vi "Teleop.vi"(10 "Match Info":T3={"Autonomous Elapsed Seconds"=0.0, "TeleOp Elapsed Seconds"=0.0, "Disabled Elapsed Seconds"=0.0, "Visited Autonomous"=FALSE, "Visited TeleOp"=FALSE, "Visited Disabled"=FALSE, "Autonomous Settings"={"Autonomous Style"=enum."Independent", "VI Refnum"=refnum}}, 11 "Call Context":T4) -> ()   [LabVIEW 2014]
doc: "This VI is called for each TeleOp packet received from the DS where the robot is not disabled. It is often used to read from the joysticks and update I/O or to update setpoints for timed control loops. It should complete and return within 20 milliseconds or it may miss DS packets."
uses:
  <vilib>/Rock Robotics/WPI/DriverStation/WPI_DriverStationDerivedRobotMode.ctl
  <vilib>/Rock Robotics/WPI/DriverStation/WPI_DriverStationMatch Info.ctl
  <vilib>/Rock Robotics/WPI/CAN/TalonSRX/WPI_CANTalonSRX_APIControlMode.ctl
  <vilib>/Rock Robotics/Network Tables/SD Write Boolean.vi
  <vilib>/Rock Robotics/Network Tables/SD Read Boolean.vi
  <vilib>/Rock Robotics/Network Tables/SD Read Number.vi
  <vilib>/Rock Robotics/WPI/Joystick/WPI_JoystickGetSetRefNum.vi
panel:
  out "ej Distance":dbl
  out "ej Rate":dbl
  out "Time elapsed":u64
  in  "Set Timer":bool
  out "cluster":T1
  out "Btm lim val":bool
  out "top lim val":bool
  out "Toggled Boolean":bool
  out "axes":T2
  out "Sample Slider 0":dbl(slide) scale=0.0..5.0
  out "Sample Boolean 1":bool
  out "Sample Boolean 0":bool
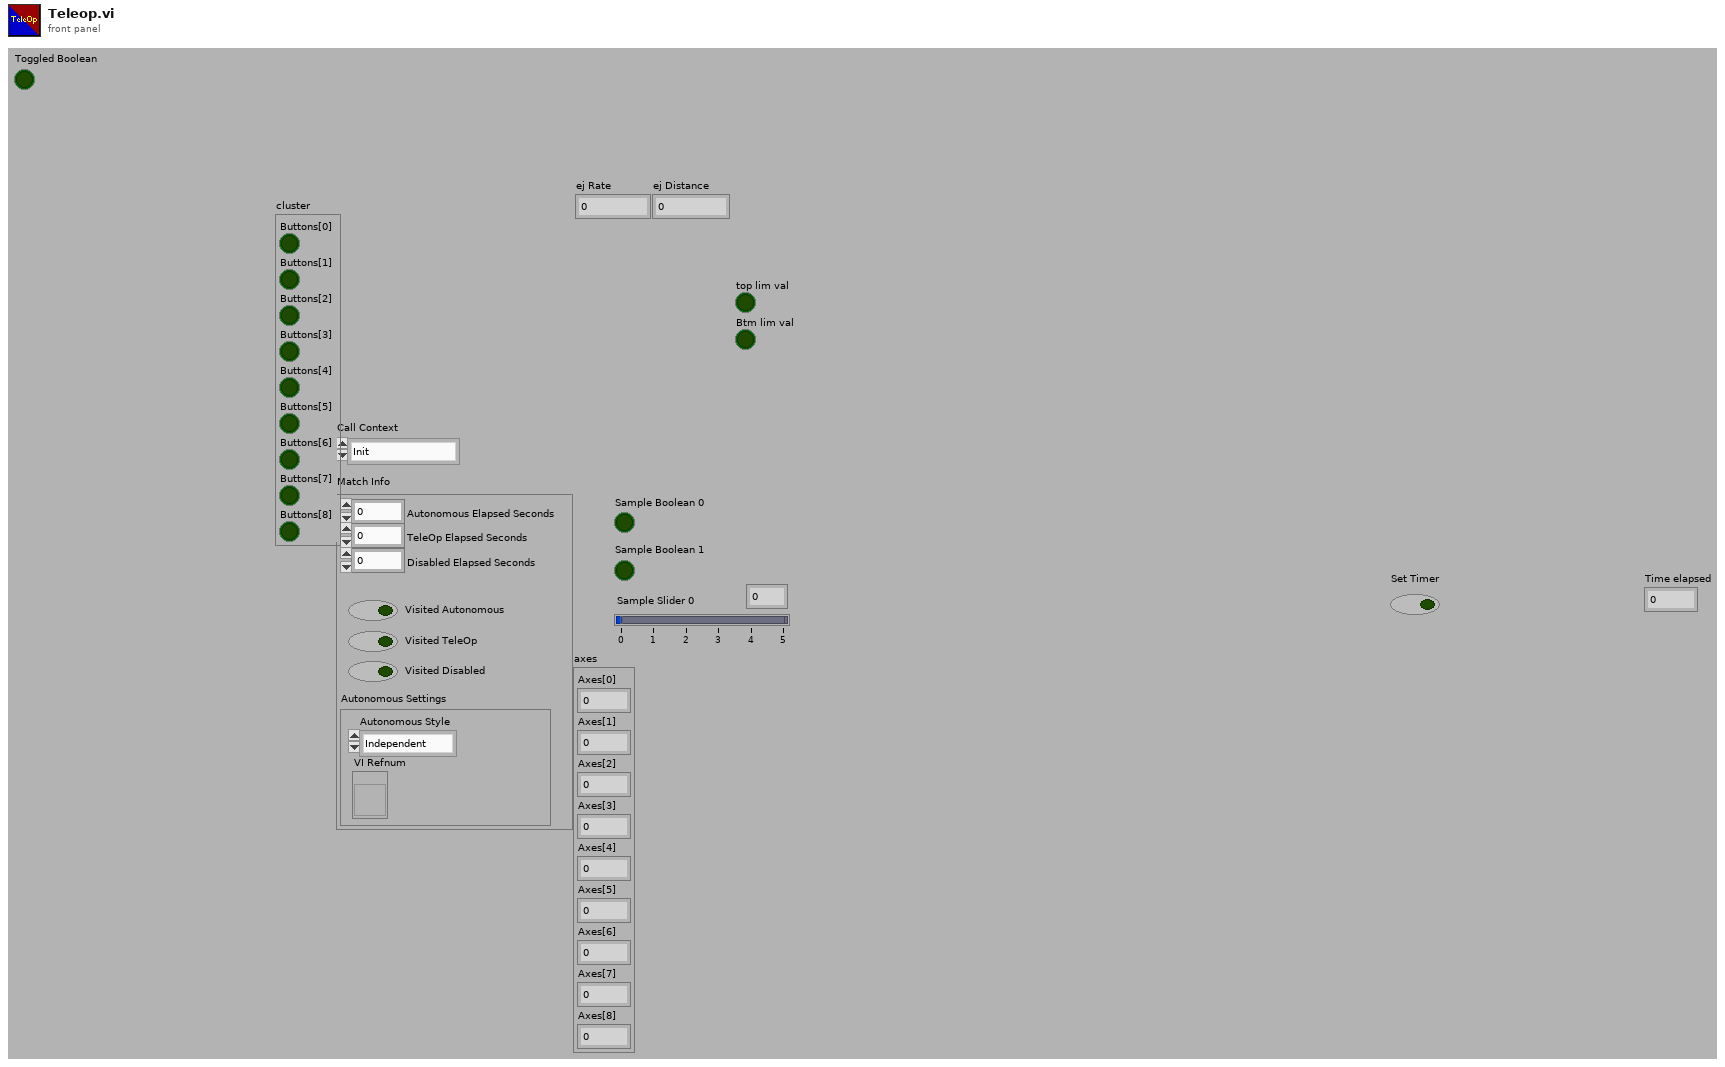
[diagram p1: front panel]
types:
  T1 = cluster{"Buttons[0]":bool, "Buttons[1]":bool, "Buttons[2]":bool, "Buttons[3]":bool, "Buttons[4]":bool, "Buttons[5]":bool, "Buttons[6]":bool, "Buttons[7]":bool, "Buttons[8]":bool}
  T2 = cluster{"Axes[0]":dbl, "Axes[1]":dbl, "Axes[2]":dbl, "Axes[3]":dbl, "Axes[4]":dbl, "Axes[5]":dbl, "Axes[6]":dbl, "Axes[7]":dbl, "Axes[8]":dbl}
  T3 = typedef "WPI_DriverStationMatch Info.ctl" = cluster{"Autonomous Elapsed Seconds":dbl, "TeleOp Elapsed Seconds":dbl, "Disabled Elapsed Seconds":dbl, "Visited Autonomous":bool, "Visited TeleOp":bool, "Visited Disabled":bool, "Autonomous Settings":cluster{"Autonomous Style":enum16{"Iterative", "Independent"}, "VI Refnum":refnum<vi>}}
  T4 = typedef "WPI_DriverStationDerivedRobotMode.ctl" = enum16{"Init", "Execute", "Stop"}
  T5 = typedef "WPI_JoystickDevRef.ctl" = cluster{"Device":T6}
  T6 = typedef "WPI_JoystickDeviceEnum.ctl" = enum16{"USB 0", "USB 1", "USB 2", "USB 3", "USB 4", "USB 5"}
  T7 = typedef "WPI_EncoderDevRef.ctl" = cluster{"DevStatus":errorcluster, "EncoderIndex":T8, "CounterIndex":T9, "DistancePerCount":dbl, "Decoding Type":T10}
  T8 = typedef "FPGA_EncoderIdx.ctl" = enum8{"Enc 0", "Enc 1", "Enc 2", "Enc 3", "Enc 4", "Enc 5", "Enc 6", "Enc 7", "Invalid"}
  T9 = typedef "FPGA_CounterCtrSystemIndex.ctl" = enum8{"Ctr 0", "Ctr 1", "Ctr 2", "Ctr 3", "Ctr 4", "Ctr 5", "Ctr 6", "Ctr 7", "Invalid"}
  T10 = typedef "WPI_EncoderType.ctl" = enum16{"1x", "2x", "4x"}
  T11 = typedef "WPI_DigitalInputDevRef.ctl" = cluster{"DevStatus":errorcluster, "DIO Channel":T12, "Controller":T13}
  T12 = typedef "FPGA_DIOChannel.ctl" = enum8{"DIO 0", "DIO 1", "DIO 2", "DIO 3", "DIO 4", "DIO 5", "DIO 6", "DIO 7", "DIO 8", "DIO 9", "DIO MXP 0", "DIO MXP 1", "DIO MXP 2", "DIO MXP 3", "DIO MXP 4", "DIO MXP 5", "DIO MXP 6", "DIO MXP 7", "DIO MXP 8", "DIO MXP 9", "DIO MXP 10", "DIO MXP 11", "DIO MXP 12", "DIO MXP 13", "DIO MXP 14", "DIO MXP 15", "Invalid"}
  T13 = typedef "FPGA_TypedefDigitalModule.ctl" = enum16{"Controller 1"}
  T14 = typedef "WPI_CANTalonSRX_APIControlMode.ctl" = enum8{"Percent VBus", "Speed", "Position", "Slave", "Unchanged / Invalid"}
  T15 = typedef "WPI_MotorControlDeviceRef.ctl" = cluster{"DeviceStatus":errorcluster, "Type":T16, "PWM":cluster{"Controller":T13, "PWM Channel":T17, "DeadBand":T18}, "CAN":cluster{"Device Number":u8, "Control Mode":T19, "Semaphore":T20, "Max Vout":dbl, "TalonSRX Control Mode":T14}, "Invert":bool, "TransformRef":T21, "InvTransformRef":T21}
  T16 = typedef "WPI_MotorControlType.ctl" = enum16{"PWM", "CAN", "CANTalonSRX"}
  T17 = typedef "FPGA_DIOPWMChannel.ctl" = enum8{"PWM 0", "PWM 1", "PWM 2", "PWM 3", "PWM 4", "PWM 5", "PWM 6", "PWM 7", "PWM 8", "PWM 9", "PWM MXP 0", "PWM MXP 1", "PWM MXP 2", "PWM MXP 3", "PWM MXP 4", "PWM MXP 5", "PWM MXP 6", "PWM MXP 7", "PWM MXP 8", "PWM MXP 9", "Invalid"}
  T18 = typedef "WPI_PWMDeadband.ctl" = cluster{"Name":string, "maxPositivePwm":i32, "minPositivePwm":i32, "centerPwm":i32, "maxNegativePwm":i32, "minNegativePwm":i32, "angularRange":u16}
  T19 = typedef "WPI_CANJaguar_ControlMode.ctl" = enum8{"Percent VBus", "Current", "Speed", "Position", "Voltage"}
  T20 = typedef "Semaphore RefNum" = refnum<k1>
  T21 = typedef "WPI_PWMTransform_ConPane.ctl" = refnum<vi>
  T22 = typedef "WPI_ServoDeviceRef.ctl" = cluster{"DeviceStatus":errorcluster, "Controller":T13, "PWM Channel":T17, "DeadBand":T18}
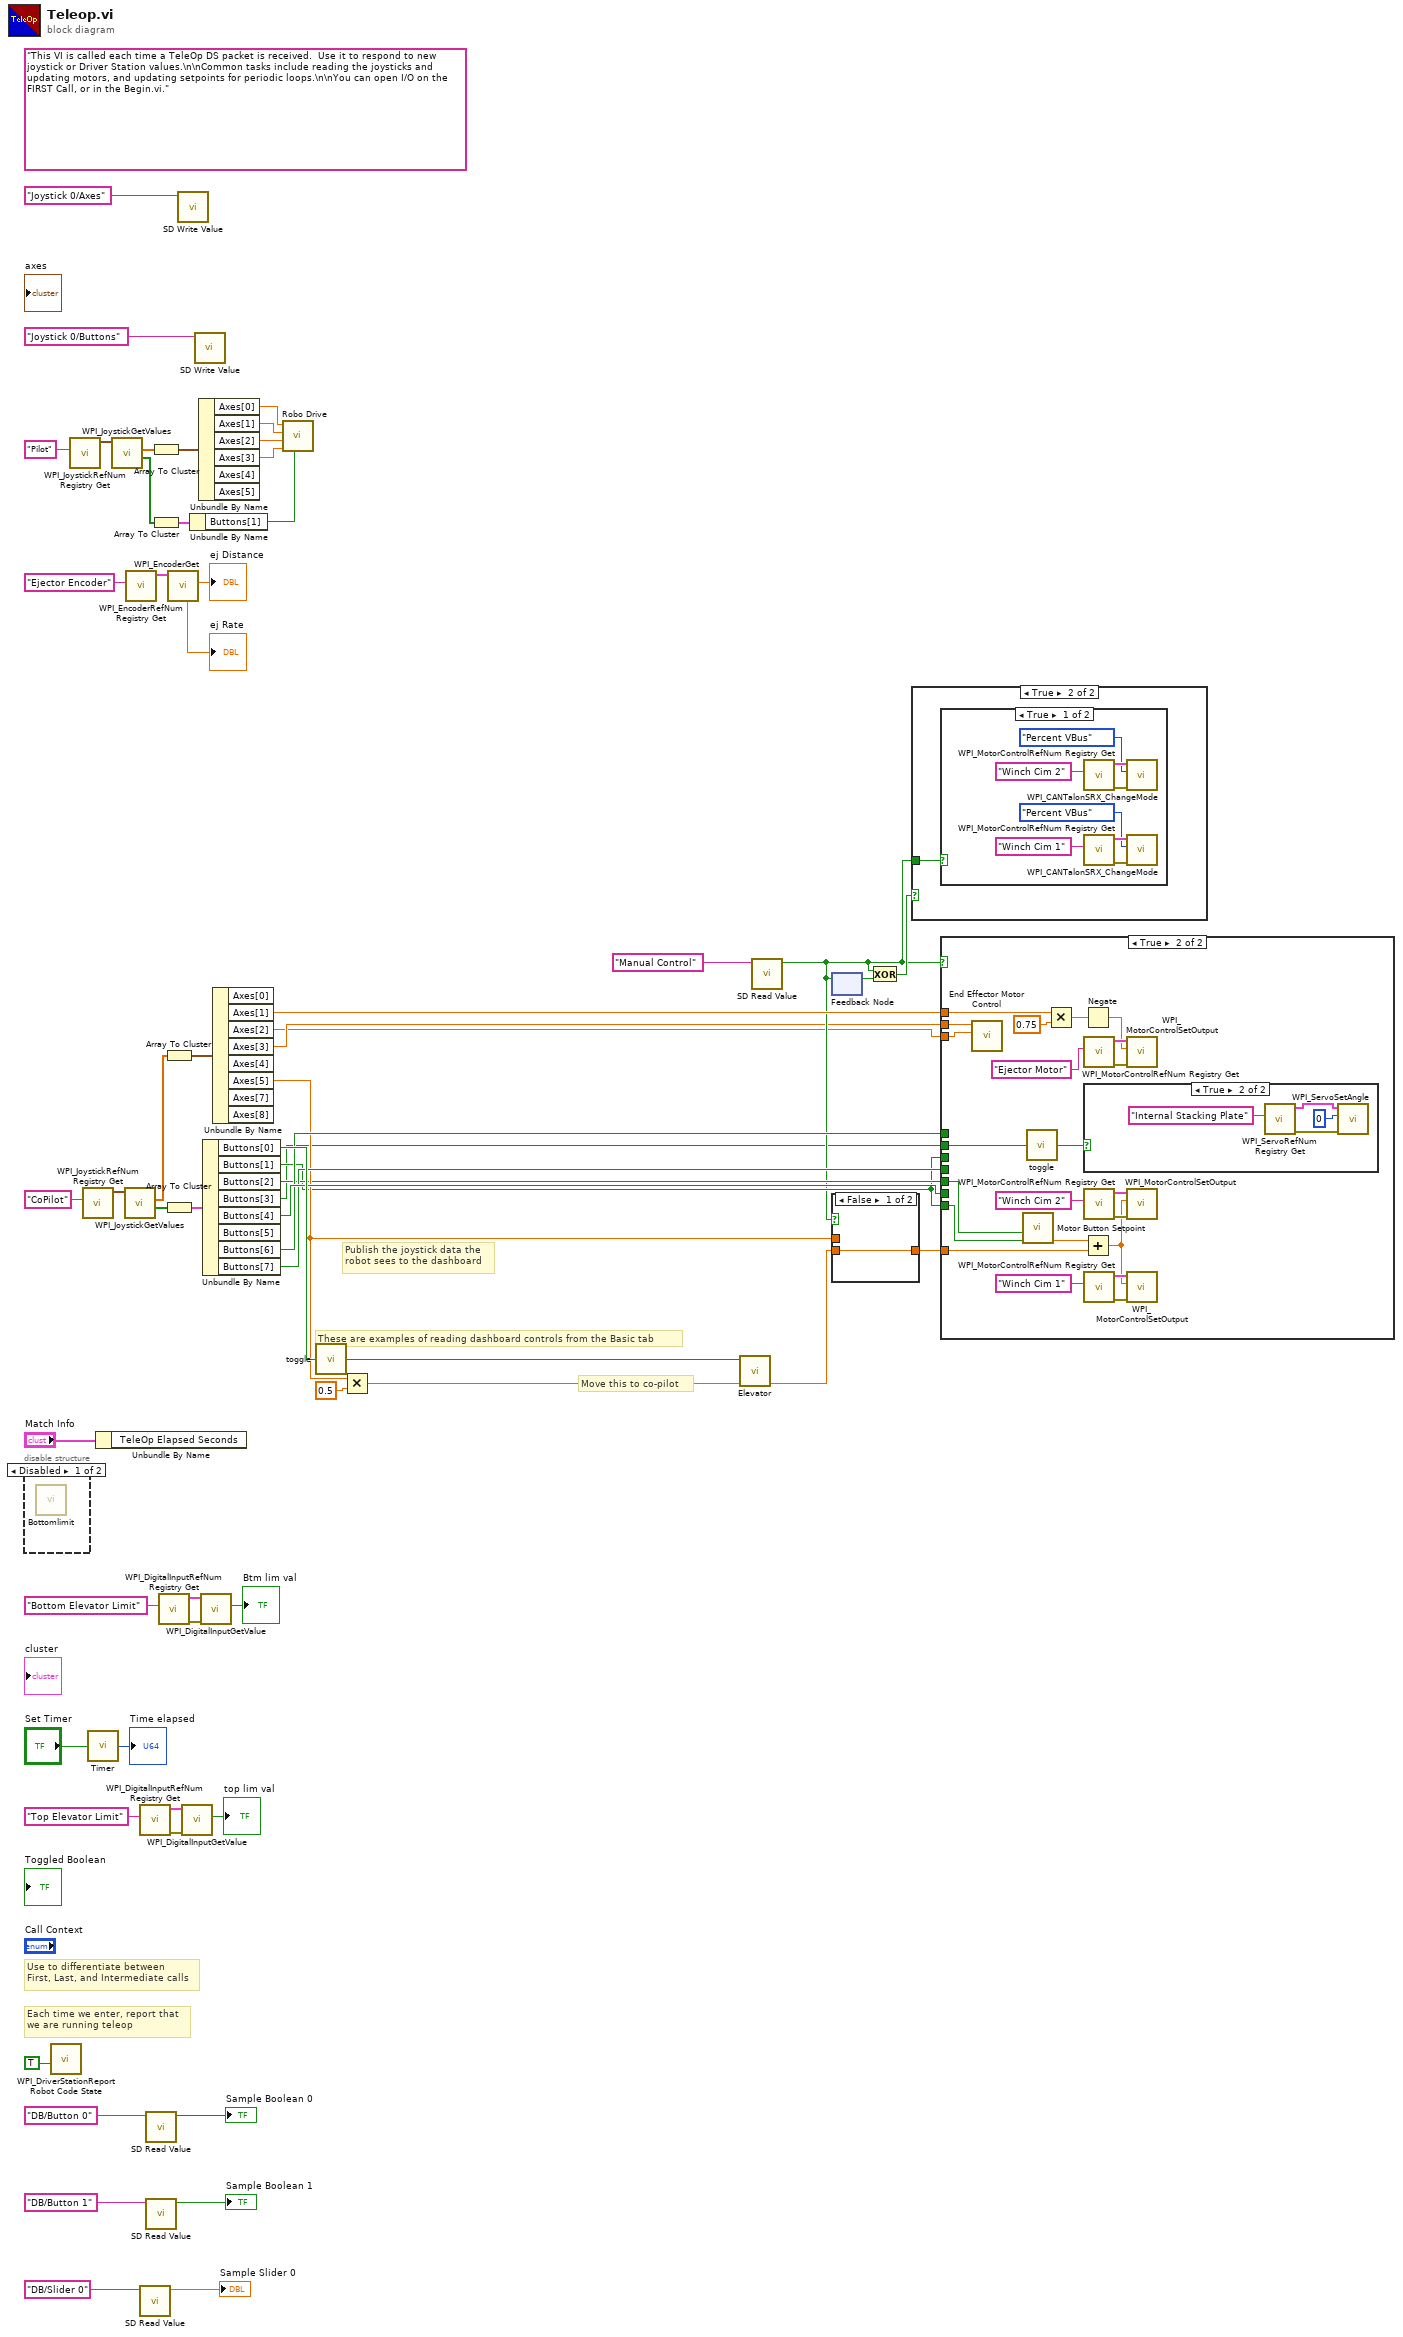
[diagram p0: block diagram]
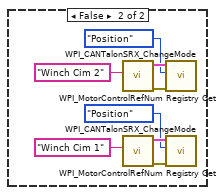
[diagram p4: hidden frame]
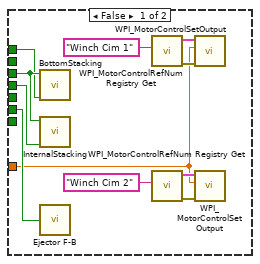
[diagram p5: hidden frame]
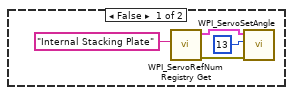
[diagram p6: hidden frame]
diagram:
  (unwired) "This VI is called each time a TeleOp DS packet is received.  Use it to respond to new joystick or Driver Station values.\n\nCommon tasks include reading the joysticks and updating motors, and updating setpoints for periodic loops.\n\nYou can open I/O on the FIRST Call, or in the Begin.vi."
  # "Move this to co-pilot"
  # "These are examples of reading dashboard controls from the Basic tab"
  # "Publish the joystick data the\nrobot sees to the dashboard"
  # "Each time we enter, report that\nwe are running teleop"
  # "Use to differentiate between\nFirst, Last, and Intermediate calls"
  n1 = disable-structure shown="Disabled" {
    frame Disabled {
      n2 = call "Bottomlimit.vi"() -> ()  [unwired: 12 in]
    }
    frame Enabled {
    }
  }
  n3 = call <vilib>:"WPI_DriverStationReport Robot Code State.vi"("TeleOp"=TRUE ("Autonomous")) -> ()  [unwired: 10 in, 1 out]
  n4 = call <vilib>:"WPI_JoystickRefNum Registry Get.vi"("refnum name"="Pilot") -> ("JoystickDevRef"=w41:T5)  [unwired: 1 in, 9 out]
  n5 = call <vilib>:"WPI_JoystickRefNum Registry Get.vi"("refnum name"="CoPilot") -> ("JoystickDevRef"=w22:T5)  [unwired: 1 in, 9 out]
  n6 = call "Timer.vi"("Set Timer"="Set Timer") -> ("Time elapsed"=→"Time elapsed":u64)
  n7 = Unbundle By Name("Match Info") -> ()  [unwired: 1 out]
  n8 = call <vilib>:"WPI_JoystickGetValues.vi"("JoystickDevRef"=w41) -> ("Buttons"=w33:bool[], "Axes"=w39:dbl[])  [unwired: 6 in, 3 out]
  n9 = call <vilib>:"WPI_JoystickGetValues.vi"("JoystickDevRef"=w22) -> ("Buttons"=w16:bool[], "Axes"=w20:dbl[])  [unwired: 6 in, 3 out]
  n10 = call <vilib>:"WPI_EncoderRefNum Registry Get.vi"("refnum name"="Ejector Encoder") -> ("EncoderDevRef"=w29:T7)  [unwired: 9 in, 1 out]
  n11 = call <vilib>:"WPI_DigitalInputRefNum Registry Get.vi"("refnum name"="Top Elevator Limit") -> ("error out"=w51:errorcluster, "DigitalInputDevRef"=w50:T11)  [unwired: 9 in]
  n12 = call-poly <vilib>:"SD Read Value.vi"("Name"="DB/Slider 0" ("refnum name")) -> ("Numeric"=→"Sample Slider 0":dbl)  [unwired: 8 in, 2 out]
  n13 = call-poly <vilib>:"SD Read Value.vi"("Name"="DB/Button 0" ("refnum name")) -> ("Boolean"=→"Sample Boolean 0":bool)  [unwired: 8 in, 2 out]
  n14 = call-poly <vilib>:"SD Read Value.vi"("Name"="DB/Button 1" ("refnum name")) -> ("Boolean"=→"Sample Boolean 1":bool)  [unwired: 8 in, 2 out]
  n15 = Array To Cluster(array=w39) -> (cluster=w38:T2)
  n16 = Array To Cluster(array=w33) -> (cluster=w32:T1)
  n17 = call <vilib>:"WPI_DigitalInputRefNum Registry Get.vi"("refnum name"="Bottom Elevator Limit") -> ("error out"=w47:errorcluster, "DigitalInputDevRef"=w46:T11)  [unwired: 9 in]
  n18 = Array To Cluster(array=w20) -> (cluster=w17:T2)
  n19 = Array To Cluster(array=w16) -> (cluster=w19:T1)
  n20 = call <vilib>:"WPI_EncoderGet.vi"("EncoderDevRef"=w29) -> ("Distance"=→"ej Distance":dbl, "Rate"=→"ej Rate":dbl)  [unwired: 5 in, 4 out]
  n21 = call-poly <vilib>:"SD Write Value.vi"("Name"="Joystick 0/Axes") -> ()  [unwired: 9 in, 2 out]
  n22 = call <vilib>:"WPI_DigitalInputGetValue.vi"("error in (no error)"=w51, "DigitalInputDevRef"=w50) -> ("Value"=→"top lim val":bool)  [unwired: 7 in, 2 out]
  n23 = Unbundle By Name(w32) -> ("Buttons[1]"=w31:bool)
  n24 = call-poly <vilib>:"SD Write Value.vi"("Name"="Joystick 0/Buttons") -> ()  [unwired: 9 in, 2 out]
  n25 = Unbundle By Name(w38) -> ("Axes[0]"=w37:dbl, "Axes[1]"=w36:dbl, "Axes[2]"=w35:dbl, "Axes[3]"=w34:dbl)  [unwired: 2 out]
  n26 = call <vilib>:"WPI_DigitalInputGetValue.vi"("error in (no error)"=w47, "DigitalInputDevRef"=w46) -> ("Value"=→"Btm lim val":bool)  [unwired: 7 in, 2 out]
  n27 = Unbundle By Name(w19) -> ("Buttons[0]"=w18:bool, "Buttons[1]"=w5:bool, "Buttons[2]"=w6:bool, "Buttons[3]"=w3:bool, "Buttons[4]"=w15:bool, "Buttons[6]"=w13:bool, "Buttons[7]"=w14:bool)  [unwired: 1 out]
  n28 = Unbundle By Name(w17) -> ("Axes[1]"=w12:dbl, "Axes[2]"=w1:dbl, "Axes[3]"=w2:dbl, "Axes[5]"=w9:dbl)  [unwired: 4 out]
  n29 = call "Robo Drive.vi"("Button Flip Directions"=w31, "Right Analog (axes 3)"=w34, "Left Analog (axes 2)"=w35, "Axes 1 (y axis)"=w36, "Axes 0 (x axis)"=w37) -> ()  [unwired: 7 in]
  n30 = call "toggle.vi"("Input"=w18) -> ("Output"=w24:bool)
  n31 = Multiply(x=w9, y=0.5) -> (x*y=w26:dbl)
  n32 = call "Elevator.vi"("actuating axis"=w26, "Elevator Locked?"=w24) -> ("Winch Setpoint"=w7:dbl)  [unwired: 9 in]
  n33 = call-poly <vilib>:"SD Read Value.vi"("Name"="Manual Control") -> ("Boolean"=w4:bool)  [unwired: 8 in, 2 out]
  n34 = feedback-in #1(w4) -> ()
  n35 = feedback #1() -> (w11:bool)  [unwired: 1 in]
  n36 = case shown="False" w4 {
    tunnel: w9 -> [_ w63]
    tunnel: [w62 w63] -> w8
    tunnel: w7 -> [w62 _]
    frame False {
    }
    frame True {
    }
  }
  n37 = Exclusive Or(1:w11, 2:w4) -> (0:w10:bool)
  n38 = case shown="True" w10 {
    tunnel: w4 -> [_ w64]
    frame False {
    }
    frame True {
      n39 = case shown="True" w64 {
        frame True {
          n40 = call <vilib>:"WPI_MotorControlRefNum Registry Get.vi"("refnum name"="Winch Cim 2") -> ("error out"=w68:errorcluster, "MotorControlDevRef"=w67:T15)  [unwired: 9 in]
          n41 = call <vilib>:"WPI_MotorControlRefNum Registry Get.vi"("refnum name"="Winch Cim 1") -> ("error out"=w72:errorcluster, "MotorControlDevRef"=w71:T15)  [unwired: 9 in]
          n42 = call <vilib>:"WPI_CANTalonSRX_ChangeMode.vi"("error in (no error)"=w68, "Control Mode"=WPI_CANTalonSRX_APIControlMode."Percent VBus", "CAN Talon SRX Ref"=w67) -> ()  [unwired: 7 in, 2 out]
          n43 = call <vilib>:"WPI_CANTalonSRX_ChangeMode.vi"("error in (no error)"=w72, "Control Mode"=WPI_CANTalonSRX_APIControlMode."Percent VBus", "CAN Talon SRX Ref"=w71) -> ()  [unwired: 7 in, 2 out]
        }
        frame False {
          n44 = call <vilib>:"WPI_MotorControlRefNum Registry Get.vi"("refnum name"="Winch Cim 2") -> ("error out"=w76:errorcluster, "MotorControlDevRef"=w75:T15)  [unwired: 9 in]
          n45 = call <vilib>:"WPI_MotorControlRefNum Registry Get.vi"("refnum name"="Winch Cim 1") -> ("error out"=w80:errorcluster, "MotorControlDevRef"=w79:T15)  [unwired: 9 in]
          n46 = call <vilib>:"WPI_CANTalonSRX_ChangeMode.vi"("error in (no error)"=w76, "Control Mode"=WPI_CANTalonSRX_APIControlMode."Position", "CAN Talon SRX Ref"=w75) -> ()  [unwired: 7 in, 2 out]
          n47 = call <vilib>:"WPI_CANTalonSRX_ChangeMode.vi"("error in (no error)"=w80, "Control Mode"=WPI_CANTalonSRX_APIControlMode."Position", "CAN Talon SRX Ref"=w79) -> ()  [unwired: 7 in, 2 out]
        }
      }
    }
  }
  n48 = case shown="True" w4 {
    tunnel: w15 -> [w91 _]
    tunnel: w5 -> [w90 _]
    tunnel: w14 -> [w89 _]
    tunnel: w13 -> [w88 _]
    tunnel: w12 -> [_ w107]
    tunnel: w8 -> [w81 w100]
    tunnel: w6 -> [_ w97]
    tunnel: w5 -> [_ w96]
    tunnel: w3 -> [_ w94]
    tunnel: w2 -> [_ w93]
    tunnel: w1 -> [_ w92]
    frame False {
      n49 = call "BottomStacking.vi"("Activating Button"=w88, "Cancel Button"=w90) -> ()  [unwired: 10 in]
      n50 = call "InternalStacking.vi"("Initialize Internal Stacking"=w89, "Cancel Internal Stacking"=w90) -> ()  [unwired: 10 in]
      n51 = call "Ejector F-B.vi"("Run Forward"=w91) -> ()  [unwired: 1 out]
      n52 = call <vilib>:"WPI_MotorControlRefNum Registry Get.vi"("refnum name"="Winch Cim 1") -> ("error out"=w86:errorcluster, "MotorControlDevRef"=w85:T15)  [unwired: 9 in]
      n53 = call <vilib>:"WPI_MotorControlRefNum Registry Get.vi"("refnum name"="Winch Cim 2") -> ("error out"=w83:errorcluster, "MotorControlDevRef"=w82:T15)  [unwired: 9 in]
      n54 = call <vilib>:"WPI_MotorControlSetOutput.vi"("error in (no error)"=w86, "Output"=w81, "MotorControlDevRef"=w85) -> ()  [unwired: 6 in, 3 out]
      n55 = call <vilib>:"WPI_MotorControlSetOutput.vi"("error in (no error)"=w83, "Output"=w81, "MotorControlDevRef"=w82) -> ()  [unwired: 6 in, 3 out]
    }
    frame True {
      n56 = call "End Effector Motor Control.vi"("Analog Input (closing)"=w92, "Analog Input (opening)"=w93) -> ()  [unwired: 10 in]
      n57 = call "Motor Button Setpoint.vi"("Subtract"=w96, "ADD"=w97) -> ("Speed"=w99:dbl)  [unwired: 9 in]
      n58 = call "toggle.vi"("Input"=w94) -> ("Output"=w95:bool)
      n59 = Multiply(x=w107, y=0.75) -> (x*y=w109:dbl)
      n60 = Negate(x=w109) -> (-x=w110:dbl)
      n61 = Add(x=w99, y=w100) -> (x+y=w98:dbl)
      n62 = call <vilib>:"WPI_MotorControlRefNum Registry Get.vi"("refnum name"="Ejector Motor") -> ("error out"=w113:errorcluster, "MotorControlDevRef"=w112:T15)  [unwired: 9 in]
      n63 = case shown="True" w95 {
        frame False {
          n64 = call <vilib>:"WPI_ServoRefNum Registry Get.vi"("refnum name"="Internal Stacking Plate") -> ("error out"=w116:errorcluster, "ServoDeviceRef"=w115:T22)  [unwired: 9 in]
          n65 = call <vilib>:"WPI_ServoSetAngle.vi"("error in (no error)"=w116, "Angle"=13, "ServoDeviceRef"=w115) -> ()  [unwired: 7 in, 2 out]
        }
        frame True {
          n66 = call <vilib>:"WPI_ServoRefNum Registry Get.vi"("refnum name"="Internal Stacking Plate") -> ("error out"=w120:errorcluster, "ServoDeviceRef"=w119:T22)  [unwired: 9 in]
          n67 = call <vilib>:"WPI_ServoSetAngle.vi"("error in (no error)"=w120, "Angle"=0, "ServoDeviceRef"=w119) -> ()  [unwired: 7 in, 2 out]
        }
      }
      n68 = call <vilib>:"WPI_MotorControlRefNum Registry Get.vi"("refnum name"="Winch Cim 2") -> ("error out"=w102:errorcluster, "MotorControlDevRef"=w101:T15)  [unwired: 9 in]
      n69 = call <vilib>:"WPI_MotorControlRefNum Registry Get.vi"("refnum name"="Winch Cim 1") -> ("error out"=w105:errorcluster, "MotorControlDevRef"=w104:T15)  [unwired: 9 in]
      n70 = call <vilib>:"WPI_MotorControlSetOutput.vi"("error in (no error)"=w113, "Output"=w110, "MotorControlDevRef"=w112) -> ()  [unwired: 6 in, 3 out]
      n71 = call <vilib>:"WPI_MotorControlSetOutput.vi"("error in (no error)"=w102, "Output"=w98, "MotorControlDevRef"=w101) -> ()  [unwired: 6 in, 3 out]
      n72 = call <vilib>:"WPI_MotorControlSetOutput.vi"("error in (no error)"=w105, "Output"=w98, "MotorControlDevRef"=w104) -> ()  [unwired: 6 in, 3 out]
    }
  }
